vi "Write Open Loop Parameters.vi"(8 "error in (no error)":errorcluster, 9 "Low PW":dbl, 10 "High-PW":dbl, 11 "Open-Loop Setpoint in":refnum<class "Open-Loop Setpoint.lvclass">) -> (0 "error out":errorcluster, 3 "Open-Loop Setpoint out":refnum<class "Open-Loop Setpoint.lvclass">)   [LabVIEW 2020, in "Open-Loop Setpoint.lvclass"]
uses:
  Open-Loop Setpoint.lvclass
  Open-Loop Setpoint.lvclass/Open-Loop Setpoint.ctl
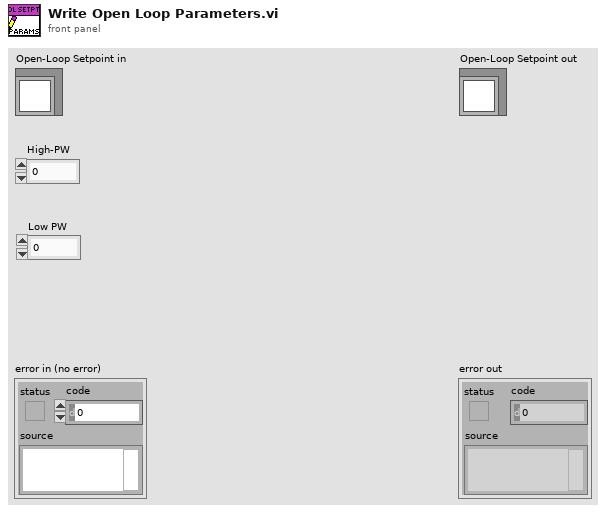
[diagram p1: front panel]
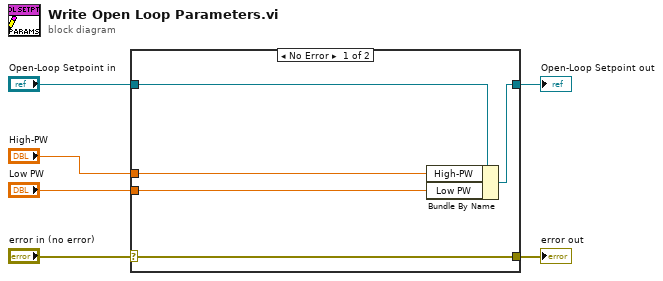
[diagram p0: block diagram]
diagram:
  n1 = case shown="No Error" "error in (no error)" {
    selector: "error in (no error)" -> [w11 w12]
    tunnel: [w11 w12] -> w5
    tunnel: [w9 w13] -> w3
    tunnel: "Open-Loop Setpoint in" -> [w10 w13]
    tunnel: "High-PW" -> [w8 _]
    tunnel: "Low PW" -> [w7 _]
    frame No Error {
      n2 = Bundle By Name(cluster=w10, "High-PW"=w8, "Low PW"=w7) -> (w9:refnum<class "Open-Loop Setpoint.lvclass">)
    }
    frame Error {
    }
  }
  "error out" <- w5
  "Open-Loop Setpoint out" <- w3
